vi "checkError.vi"(8 "error in (no error)":errorcluster, 11 "TCPServer in":refnum<class "TCPServer.lvclass">) -> (0 "error out":errorcluster, 2 "timeout?":bool, 3 "TCPServer out":refnum<class "TCPServer.lvclass">)   [LabVIEW 2016, in "TCPServer.lvclass"]
uses:
  TCPServer.lvclass
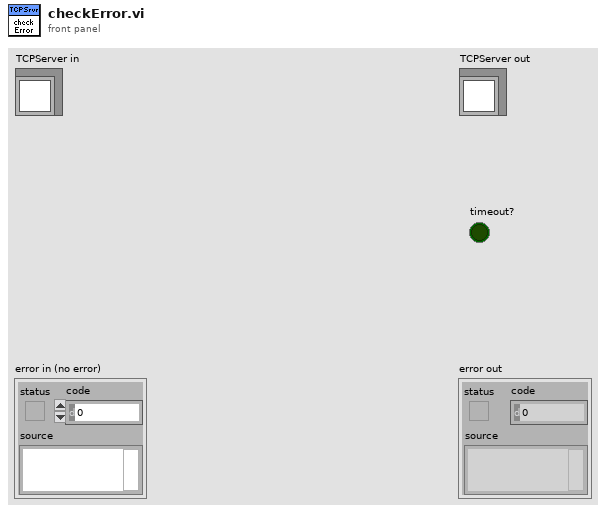
[diagram p1: front panel]
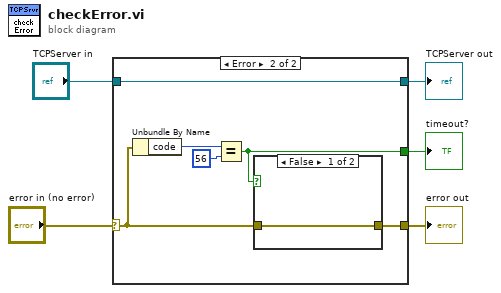
[diagram p0: block diagram]
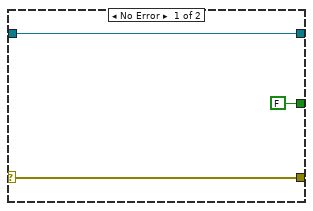
[diagram p2: hidden frame]
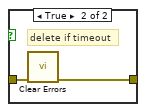
[diagram p3: hidden frame]
diagram:
  n1 = case shown="Error" "error in (no error)" {
    selector: "error in (no error)" -> [w7 w10]
    tunnel: [w7 w9] -> w4
    tunnel: [w8 w14] -> w2
    tunnel: "TCPServer in" -> [w8 w14]
    tunnel: [FALSE ("timeout?") w11] -> w1
    frame No Error {
    }
    frame Error {
      n2 = Unbundle By Name(w10) -> ("code"=w13:i32)
      n3 = Equal?(x=w13, y=56) -> (x = y?=w11:bool)
      n4 = case shown="False" w11 {
        tunnel: w10 -> [w15 w17]
        tunnel: [w15 w16] -> w9
        frame False {
        }
        frame True {
          # "delete if timeout"
          n5 = call <vilib>:"Clear Errors.vi"("error in (no error)"=w17) -> ("error out"=w16:errorcluster)  [unwired: 5 in, 1 out]
        }
      }
    }
  }
  "error out" <- w4
  "TCPServer out" <- w2
  "timeout?" <- w1
